vi "bus_monitor_server_api.CreateInstance.vi"(7 "Listening Port (0 = auto)":i32, 8 "error in (no error)":errorcluster, 10 "Name":string, 11 "IP":string) -> (0 "error out":errorcluster, 3 "gRPC Container out":refnum<class "bus_monitor_server_api.lvclass">)   [LabVIEW 2025, in "bus_monitor_server_api.lvlib" / "bus_monitor_server_api.lvclass"]
uses:
  bus_monitor_server_api.lvclass
  bus_monitor_server_api.lvclass/bus_monitor_server_api.ctl
  bus_monitor_server/RPC Service/Bus_Monitor_API/Bus_Monitor_API.lvclass
  C:/Program Files/National Instruments/LabVIEW 2025/vi.lib/gRPC/LabVIEW gRPC Servicer/ServiceBase/ServiceBase.lvclass
  C:/Projects/g/Source/Bus Monitor/Server/bus_monitor_server/RPC Service/Bus_Monitor_API/Bus_Monitor_API.lvclass
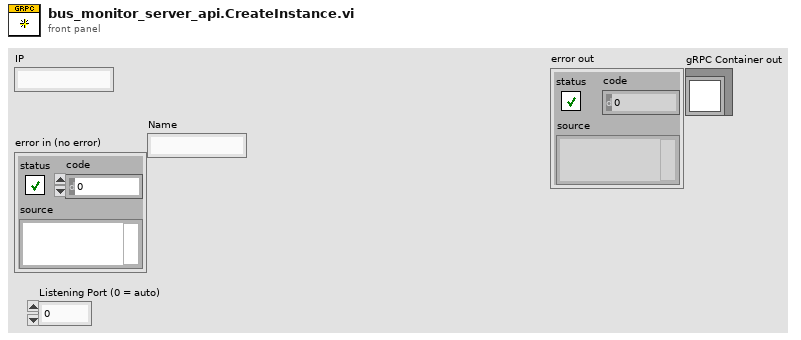
[diagram p1: front panel]
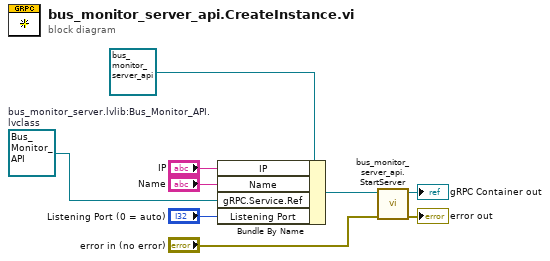
[diagram p0: block diagram]
diagram:
  w1 = refnum<class "Bus_Monitor_API.lvclass"> refnum  # bus_monitor_server.lvlib:Bus_Monitor_API.lvclass
  n1 = Bundle By Name(cluster=refnum<class "bus_monitor_server_api.lvclass"> refnum ("bus_monitor_server_api.lvlib:bus_monitor_server_api.lvclass"), "IP"="IP", "Name"="Name", "gRPC.Service.Ref"=w1, "Listening Port"="Listening Port (0 = auto)") -> (w8:refnum<class "bus_monitor_server_api.lvclass">)
  n2 = call-dynamic "bus_monitor_server_api.StartServer.vi"("error in (no error)"="error in (no error)", "gRPC Container in"=w8) -> ("error out"=→"error out":errorcluster, "gRPC Container out"=→"gRPC Container out":refnum<class "bus_monitor_server_api.lvclass">)  [unwired: 8 in]
